vi "variantCtrlSetpoint.vi"(4 "isRequired(T)":bool=TRUE, 6 "get/set":enum16{"get", "set"}(ring), 8 "error in":errorcluster, 9 "setpoint":cluster{"comparison":string, "Y":dbl}, 11 "procElement in in":variant) -> (0 "error out":errorcluster, 1 "setpoint":cluster{"Comparison":string, "Setpoint":dbl}, 2 "found/replaced":bool, 3 "procElement out":variant)   [LabVIEW 2024]
uses:
  controls/typeStepVarients.ctl
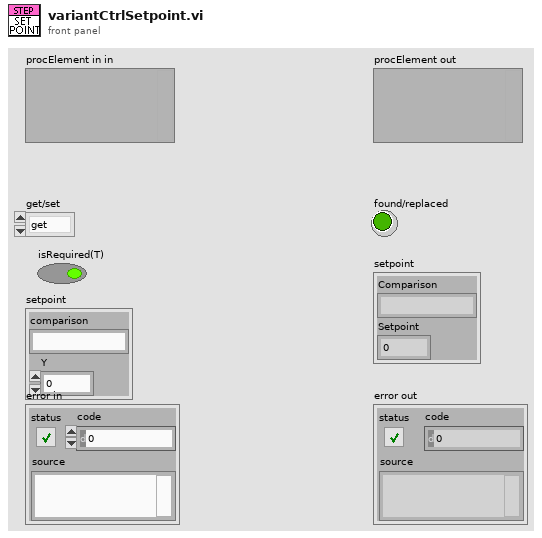
[diagram p1: front panel]
types:
  T1 = typedef "typeStepVarients.ctl" = enum16{"stepNameID", "stepFunction", "stepReport", "stepSetpoint", "stepPointer", "stepProcPointer", "stepIoPointer", "stepIoValue", "stepFilePointer", "stepMessage", "stepTimeString", "stepNumReg", "stepStrReg", "stepSeconds", "stepUnitDoseParams", "stepUnitIndex"}
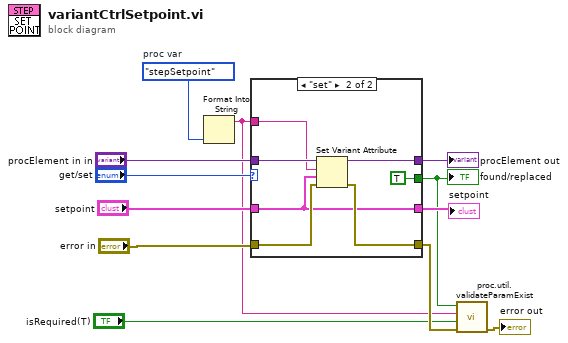
[diagram p0: block diagram]
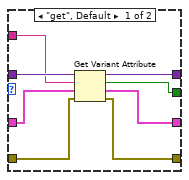
[diagram p2: hidden frame]
diagram:
  w2 = typeStepVarients."stepSetpoint"  # proc var
  n1 = Format Into String(w2) -> (resulting string=w1:string)  [unwired: 3 in, 1 out]
  n2 = case shown="\"set\"" "get/set" {
    tunnel: "procElement in in" -> [w20 w27]
    tunnel: [w19 w26] -> w8
    tunnel: [w18 TRUE] -> w6
    tunnel: "error in" -> [w16 w25]
    tunnel: [w17 w24] -> w5
    tunnel: "setpoint" -> [w14 w23]
    tunnel: [w15 w23] -> w11
    tunnel: w1 -> [w13 w22]
    frame "get", Default {
      n3 = Get Variant Attribute(Variant=w20, name=w13, default value (empty Variant)=w14, error in=w16) -> (duplicate Variant=w19:variant, found=w18:bool, value=w15:cluster{"comparison":string, "Y":dbl}, error out=w17:errorcluster)
    }
    frame "set" {
      n4 = Set Variant Attribute(Variant=w27, name=w22, value=w23, error in=w25) -> (Variant out=w26:variant, error out=w24:errorcluster)  [unwired: 1 out]
    }
  }
  "setpoint" <- w11
  "found/replaced" <- w6
  "procElement out" <- w8
  n5 = call "proc.util.validateParamExist.vi"("error in"=w5, "isRequired"="isRequired(T)", "Param Label"=w1, "isFound"=w6) -> ("error out"=→"error out":errorcluster)  [unwired: 7 in]
